vi "Simple Web Server.vi"() -> ()   [LabVIEW 2014, in "ESP8266 WiFi Wrapper.lvlib"]
uses:
  <vilib>/Aledyne-TSXperts/Arduino Compatible Compiler for LabVIEW/addons/ESP8266 WiFi Wrapper/ESP8266 WiFi Wrapper.lvlib
  <vilib>/Aledyne-TSXperts/Arduino Compatible Compiler for LabVIEW/Arduino Compatible Compiler for LabVIEW.lvlib
panel:
  in  "DNS address":u8[](array[numeric])=[1, 2, 3, 4]
  in  "IP address":u8[](array[numeric])=[192, 168, 0, 42]
  in  "Gateway":u8[](array[numeric])=[192, 168, 0, 1]
  in  "Subnet mask":u8[](array[numeric])=[255, 255, 255, 0]
  in  "Password":string="12345678"
  in  "SSID":string="ESP8266 Wifi Example"
  in  "Listen Port":u8=80
  in  "error in (no error)":errorcluster
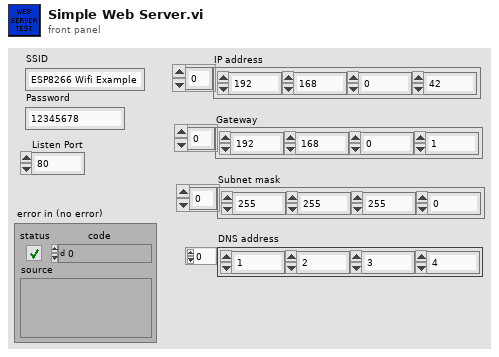
[diagram p1: front panel]
types:
  T1 = enum16{"WIFI_OFF", "WIFI_STA", "WIFI_AP", "WIFI_AP_STA"}
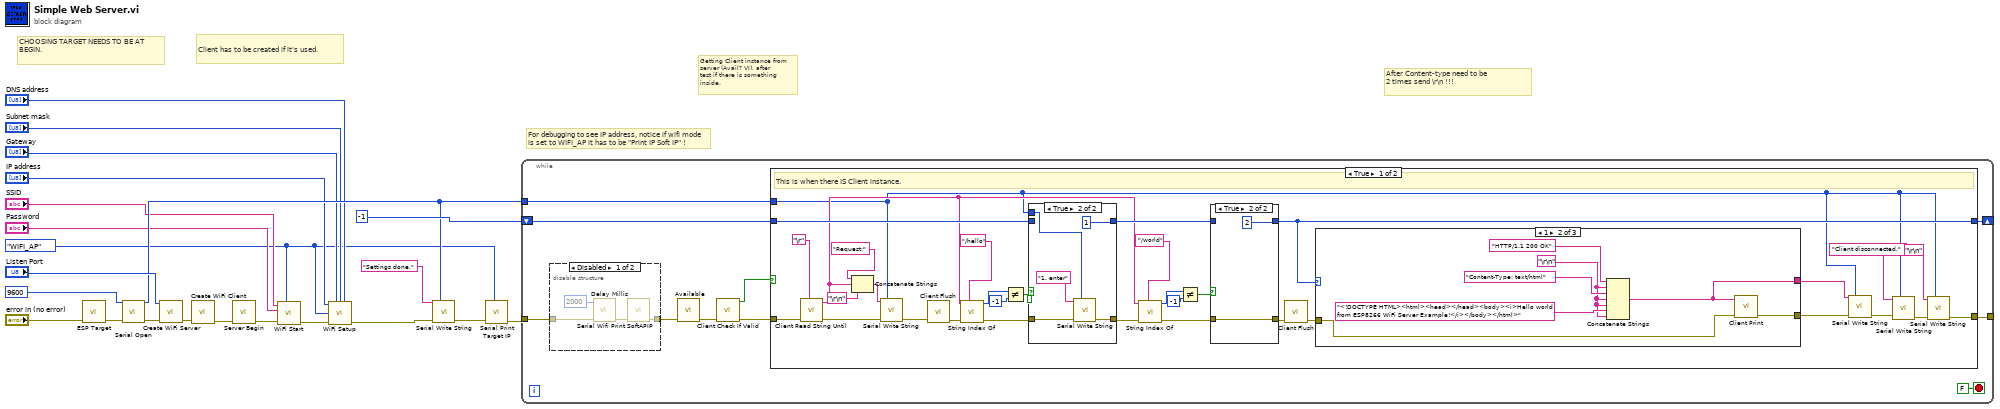
[diagram p0: block diagram]
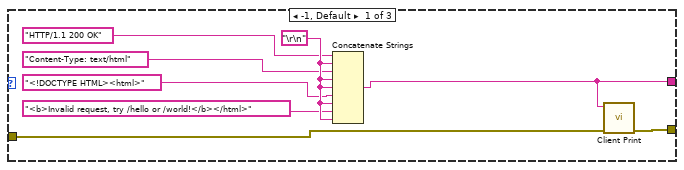
[diagram p3: hidden frame]
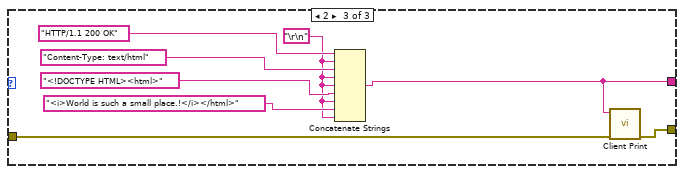
[diagram p4: hidden frame]
diagram:
  w1 = T1."WIFI_AP" ("WiFi Server Mode")
  # "For debugging to see IP address, notice if wifi mode\nis set to WIFI_AP it has to be \"Print IP Soft IP\" !"
  # "After Content-type need to be\n2 times send \\r\\n !!!"
  # "Getting Client instance from\nserver (Avail? VI), after\ntest if there is something\ninside."
  # "CHOOSING TARGET NEEDS TO BE AT BEGIN."
  # "Client has to be created if it's used."
  n1 = call <vilib>:"ESP Target.vi"("Error In"="error in (no error)") -> ("Error Out"=w17:errorcluster)  [unwired: 10 in]
  n2 = call <vilib>:"Serial Open.vi"("Speed"=u32 9600, "error in (no error)"=w17) -> ("Instance"=w15:u8, "error out"=w21:errorcluster)  [unwired: 12 in]
  n3 = call <vilib>:"Create WiFi Server.vi"("Error In"=w21, "Listen Port"="Listen Port") -> ("Error Out"=w18:errorcluster)  [unwired: 9 in]
  n4 = call <vilib>:"Create WiFi Client.vi"("Error In"=w18) -> ("Error Out"=w11:errorcluster)  [unwired: 10 in]
  n5 = call <vilib>:"Server Begin.vi"("Error In"=w11) -> ("Error Out"=w13:errorcluster)  [unwired: 10 in]
  n6 = call <vilib>:"WiFi Start.vi"("WiFi Mode"=w1, "Error In"=w13, "Password"="Password", "SSID"="SSID") -> ("Error Out"=w12:errorcluster)  [unwired: 7 in]
  n7 = call <vilib>:"WiFi Setup.vi"("IP address"="IP address", "Gateway address"="Gateway", "Subnet mask"="Subnet mask", "DNS address"="DNS address", "WiFi Mode"=w1, "Error In"=w12) -> ("Error Out"=w10:errorcluster)  [unwired: 9 in]
  n8 = call <vilib>:"Serial Write String.vi"("String"="Settings done.", "Instance"=w15, "error in (no error)"=w10) -> ("error out"=w3:errorcluster)  [unwired: 12 in]
  n9 = call <vilib>:"Serial Print Target IP.vi"("WiFi Mode"=w1, "Error In"=w3) -> ("Error Out"=w2:errorcluster)  [unwired: 9 in]
  n10 = while {
    tunnel: [w30] -> _
    shift-right: [w28] -> _
    shift-left: i8 -1 -> [w29]
    tunnel: w15 -> [w27]
    tunnel: w2 -> [w24]
    stop <- FALSE stop-if-true
    n11 = disable-structure shown="Disabled" {
      disable-tunnel: [w36 w37] -> w25
      disable-tunnel: w24 -> [w33 w37]
      frame Disabled {
        n12 = call <vilib>:"Delay Millis.vi"("error in (no error)"=w33, "delay"=u32 2000) -> ("error out"=w34:errorcluster)  [unwired: 9 in]
        n13 = call <vilib>:"Serial Wifi Print SoftAPIP.vi"("Error In"=w34) -> ("Error Out"=w36:errorcluster)  [unwired: 10 in]
      }
      frame Enabled {
      }
    }
    n14 = call <vilib>:"Available.vi"("Error In"=w25) -> ("Error Out"=w23:errorcluster)  [unwired: 10 in]
    n15 = call <vilib>:"Client Check If Valid.vi"("Error In"=w23) -> ("Error Out"=w26:errorcluster, "Is Null?"=w31:bool)  [unwired: 9 in]
    n16 = case shown="True" w31 {
      tunnel: w26 -> [w70 w106]
      tunnel: [w46 w106] -> w30
      tunnel: [w53 w105] -> w28
      tunnel: w29 -> [w56 w105]
      tunnel: w27 -> [w40 _]
      frame True {
        # "This is when there IS Client instance."
        n17 = call <vilib>:"Client Read String Until.vi"("Terminator char"="\r" ("Carriage Return Constant"), "Error In"=w70) -> ("Error Out"=w51:errorcluster, "Read String"=w43:string)  [unwired: 8 in]
        n18 = Concatenate Strings("Request:" ("string"), w43, "\r\n" ("End of Line Constant")) -> (w45:string)
        n19 = call <vilib>:"Serial Write String.vi"("String"=w45, "Instance"=w40, "error in (no error)"=w51) -> ("error out"=w50:errorcluster)  [unwired: 12 in]
        n20 = call <vilib>:"Client Flush.vi"("Error In"=w50) -> ("Error Out"=w68:errorcluster)  [unwired: 10 in]
        n21 = call <vilib>:"String Index Of.vi"("IndexOf String"="/hello", "Error In"=w68, "Input String"=w43) -> ("Error Out"=w63:errorcluster, "index"=w66:i8)  [unwired: 7 in]
        n22 = Not Equal?(x=w66, y=i8 -1) -> (x != y?=w65:bool)
        n23 = case shown="True" w65 {
          tunnel: [w99 w103] -> w57
          tunnel: w63 -> [w99 w102]
          tunnel: [w98 i8 1] -> w55
          tunnel: w56 -> [w98 _]
          tunnel: w40 -> [_ w101]
          frame False {
          }
          frame True {
            n24 = call <vilib>:"Serial Write String.vi"("String"="1. enter", "Instance"=w101, "error in (no error)"=w102) -> ("error out"=w103:errorcluster)  [unwired: 12 in]
          }
        }
        n25 = call <vilib>:"String Index Of.vi"("IndexOf String"="/world", "Error In"=w57, "Input String"=w43) -> ("Error Out"=w62:errorcluster, "index"=w59:i8)  [unwired: 7 in]
        n26 = Not Equal?(x=w59, y=i8 -1) -> (x != y?=w60:bool)
        n27 = case shown="True" w60 {
          tunnel: [w95 w97] -> w54
          tunnel: w62 -> [w95 w97]
          tunnel: [w94 i8 2] -> w53
          tunnel: w55 -> [w94 _]
          frame False {
          }
          frame True {
          }
        }
        n28 = call <vilib>:"Client Flush.vi"("Error In"=w54) -> ("Error Out"=w52:errorcluster)  [unwired: 10 in]
        n29 = case shown="1" w53 {
          tunnel: [w77 w85 w92] -> w38
          tunnel: w52 -> [w78 w81 w93]
          tunnel: [w71 w80 w86] -> w39
          frame -1, Default {
            w76 = "\r\n" ("End of Line Constant")
            n30 = Concatenate Strings("HTTP/1.1 200 OK", w76, "Content-Type: text/html", w76, w76, "<!DOCTYPE HTML><html>", w76, "<b>Invalid request, try /hello or /world!</b></html>", w76) -> (w71:string)
            n31 = call <vilib>:"Client Print.vi"("Error In"=w78, "Input String"=w71) -> ("Error Out"=w77:errorcluster)  [unwired: 9 in]
          }
          frame 1 {
            w79 = "\r\n" ("End of Line Constant")
            n32 = Concatenate Strings("HTTP/1.1 200 OK", w79, "Content-Type: text/html", w79, w79, "<!DOCTYPE HTML><html><head></head><body><i>Hello world from ESP8266 WiFi Server Example!</i></body></html>", w79) -> (w80:string)
            n33 = call <vilib>:"Client Print.vi"("Error In"=w81, "Input String"=w80) -> ("Error Out"=w85:errorcluster)  [unwired: 9 in]
          }
          frame 2 {
            w87 = "\r\n" ("End of Line Constant")
            n34 = Concatenate Strings("HTTP/1.1 200 OK", w87, "Content-Type: text/html", w87, w87, "<!DOCTYPE HTML><html>", w87, "<i>World is such a small place.!</i></html>", w87) -> (w86:string)
            n35 = call <vilib>:"Client Print.vi"("Error In"=w93, "Input String"=w86) -> ("Error Out"=w92:errorcluster)  [unwired: 9 in]
          }
        }
        n36 = call <vilib>:"Serial Write String.vi"("String"=w39, "Instance"=w40, "error in (no error)"=w38) -> ("error out"=w41:errorcluster)  [unwired: 12 in]
        n37 = call <vilib>:"Serial Write String.vi"("String"="Client disconnected.", "Instance"=w40, "error in (no error)"=w41) -> ("error out"=w49:errorcluster)  [unwired: 12 in]
        n38 = call <vilib>:"Serial Write String.vi"("String"="\r\n" ("End of Line Constant"), "Instance"=w40, "error in (no error)"=w49) -> ("error out"=w46:errorcluster)  [unwired: 12 in]
      }
      frame False {
        # "No Client instance, do nothing."
      }
    }
  }
